vi "PH_Calorimeter_USB.ProcCases.vi"(0 "i ref in":refnum<vi>, 1 "selector":string, 2 "Data":T1, 3 "call cluster":T2={"Object"="", "Selector"="", "CallType"=enum."synchronous", "Async Object"="", "Async Selector"="", "Data Descriptor"="", "Data"=[], "Error #"=0, "Expire"=0}, 5 "error in (no error)":errorcluster) -> (14 "i ref out":refnum<vi>, 17 "answer cluster":T2={"Object"="", "Selector"="", "CallType"=enum."synchronous", "Async Object"="", "Async Selector"="", "Data Descriptor"="", "Data"=[], "Error #"=0, "Expire"=0}, 19 "error out":errorcluster)   [LabVIEW 2014, in "PH_Calorimeter_USB.lvlib"]
doc: "This method is called by a process from within the default case in the event loop. The methods of a class that are linked to events will be called from THIS method. Add your code here."
uses:
  PH_Calorimeter_USB.lvlib
  CSCore/CSSystem/CoreDefs/CoreDefs.call_type.ctl
  CSCore/BaseProcess/BaseProcess.descriptor string definition.ctl
  CSCore/CSSystem/CoreDefs/CoreDefs.rawDataType.ctl
  PH_Calorimeter_USB.Calorimeter Settings.ctl
  PH_Calorimeter_USB.Trigger Settings.ctl
  PH_Calorimeter_USB.Calorimeter Calibration Settings.ctl
  CSCore/CSSystem/CoreLib/CoreLib.byte array 2 string.vi
  CSCore/CSSystem/CoreLib/CoreLib.string 2 byte array.vi
  CSCore/CSSystem/CoreLib/CoreLib.byte array 2 double.vi
  CSCore/CSSystem/CoreLib/CoreLib.byte array 2 int.vi
  CSCore/CSSystem/CoreLib/CoreLib.lvlib
  CSCore/BaseProcess/BaseProcess.lvlib
  PH_PSDBWriter/PH_PSDBWriter.lvlib
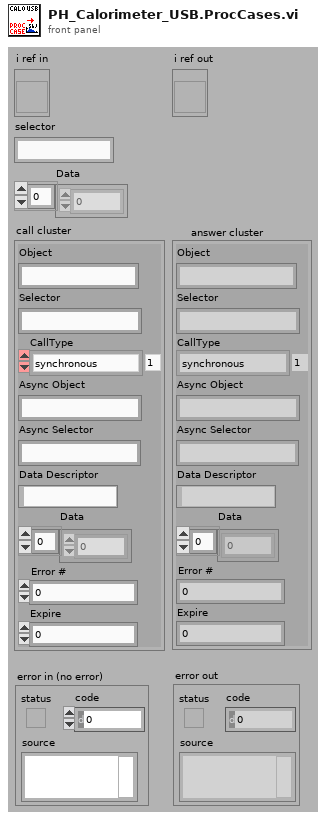
[diagram p1: front panel]
types:
  T1 = typedef "CoreDefs.rawDataType.ctl" = i8[]
  T2 = typedef "CoreDefs.call_type.ctl" = cluster{"Object":string, "Selector":string, "CallType":enum16{"simple", "synchronous", "asynchronous"}, "Async Object":string, "Async Selector":string, "Data Descriptor":T3, "Data":T1, "Error #":i32, "Expire":u32}
  T3 = typedef "BaseProcess.lvlib/BaseProcess.descriptor string definition.ctl" = string
  T4 = typedef "PH_Calorimeter_USB.lvlib/PH_Calorimeter_USB.Calorimeter Settings.ctl" = cluster{"Channel":tag, "Min Value [V]":dbl, "Max Value  [V]":dbl}
  T5 = typedef "PH_Calorimeter_USB.lvlib/PH_Calorimeter_USB.Trigger Settings.ctl" = cluster{"Channel":tag, "Min Value [V]":dbl, "Max Value  [V]":dbl, "Level [V]":dbl, "Wait Time [s]":dbl, "Length [Samples]":i32}
  T6 = typedef "PH_Calorimeter_USB.lvlib/PH_Calorimeter_USB.Calorimeter Calibration Settings.ctl" = cluster{"T 1/e [s]":dbl, "Sensitivity  [Vs/J]":dbl}
  T7 = typedef "PH_Calorimeter_USB.lvlib/PH_Calorimeter_USB.i attribute.ctl" = cluster{"GUI Refs":cluster{"Delete":refnum<vi>, "Start":refnum<vi>, "Energy":refnum<vi>, "Calorimeter":refnum<vi>, "Trigger":refnum<vi>, "Calo Calibration":refnum<vi>, "Time Base":refnum<vi>, "Device":refnum<vi>, "Graph Raw Data":refnum<vi>, "Graph Result":refnum<vi>}, "DAQ Instance":string, "Data":dbl[][], "Controller Instance":string, "Energy [J]":dbl, "Calorimeter":T4, "Trigger":T5, "Time Base":T8, "Calo Calibration":T6, "Serial Number":string}
  T8 = typedef "PH_Calorimeter_USB.lvlib/PH_Calorimeter_USB.Time Base Settings.ctl" = cluster{"Samples per Channel":i32, "Rate [Hz]":i32}
  T9 = typedef "PH_PSDBWriter.lvlib/PH_PSDBWriter.i attribute.ctl" = cluster{"PSDB Status Service ID":i32, "Instance ID":i32, "Shot #":i32, "Subsystem":T10, "Data Status":T11, "Ref PSDB Status":refnum<vi>, "PSDB Error Code":i32, "PSDB Dataset":T12, "PSDB Thread":cluster{"Ref":refnum<vi>, "Q-Ref":refnum<queue>}, "PSDB Credentials":T20}
  T10 = typedef "PH_PSDBWriter.lvlib/PH_PSDBWriter.PHELIX-Subsystems.ctl" = i32
  T11 = typedef "PH_PSDBWriter.lvlib/PH_PSDBWriter.Data Status.ctl" = i16
  T12 = typedef "PH_PSDBWriter.lvlib/PH_PSDBWriter.PSDB Dataset.ctl" = cluster{"Version":i32, "2D data Input":T13[], "Boolean Input":T15[], "Image Input":T16[], "Numeric Input":T18[], "String Input":T19[]}
  T13 = typedef "PH_PSDBWriter.lvlib/PH_PSDBWriter.2D dataset.ctl" = cluster{"name":string, "data":dbl[][], "axis description":T14}
  T14 = typedef "PSDB.lvlib/PSDB_AxisDescription.ctl" = cluster{"x axis label":string, "y axis label":string, "x axis unit":string, "y axis unit":string}
  T15 = typedef "PH_PSDBWriter.lvlib/PH_PSDBWriter.Boolean dataset.ctl" = cluster{"name":string, "data":bool, "unit":string}
  T16 = typedef "PH_PSDBWriter.lvlib/PH_PSDBWriter.Image dataset.ctl" = cluster{"name":string, "data":T17, "unit":string}
  T17 = typedef "IMAQ Image.ctl" = refnum<image>
  T18 = typedef "PH_PSDBWriter.lvlib/PH_PSDBWriter.Numeric dataset.ctl" = cluster{"name":string, "data":dbl, "unit":string}
  T19 = typedef "PH_PSDBWriter.lvlib/PH_PSDBWriter.String dataset.ctl" = cluster{"name":string, "data":string, "unit":string}
  T20 = typedef "PH_Common.lvlib/PH_Connection.PSDB Credentials.ctl" = cluster{"PW":string, "ID":string, "DS":string}
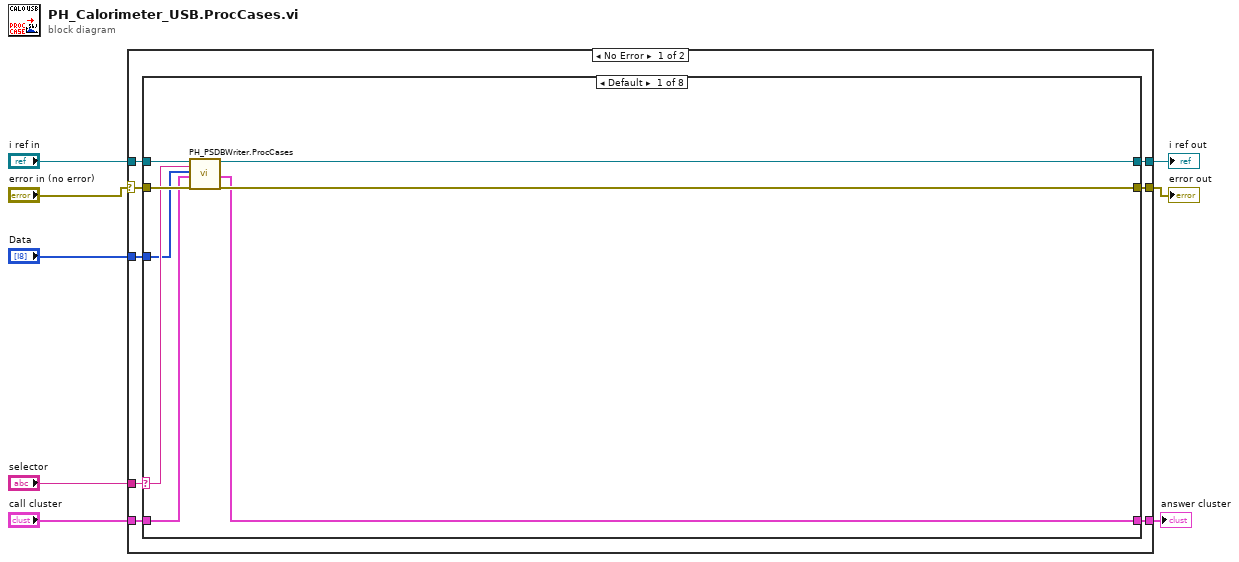
[diagram p0: block diagram]
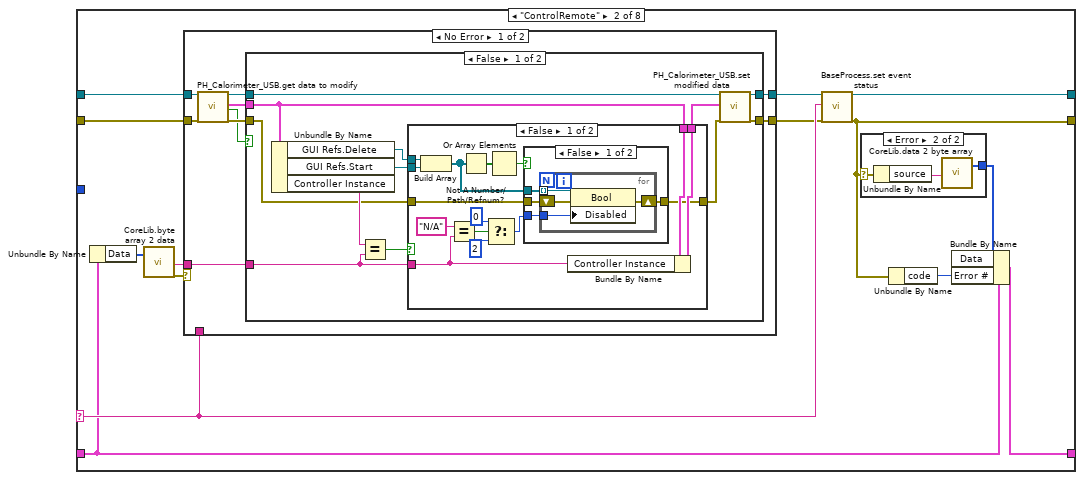
[diagram p2: hidden frame]
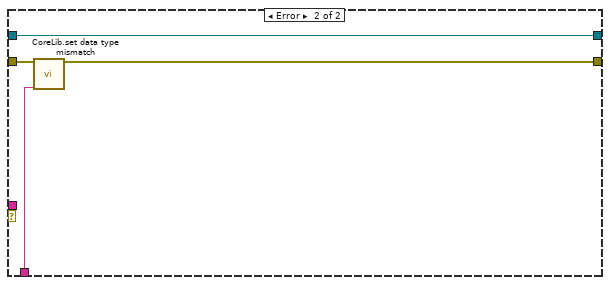
[diagram p7: hidden frame]
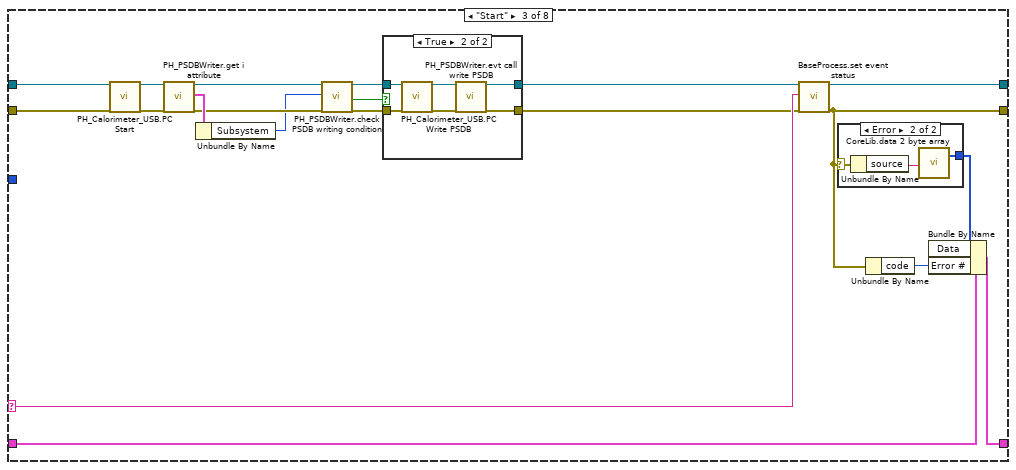
[diagram p8: hidden frame]
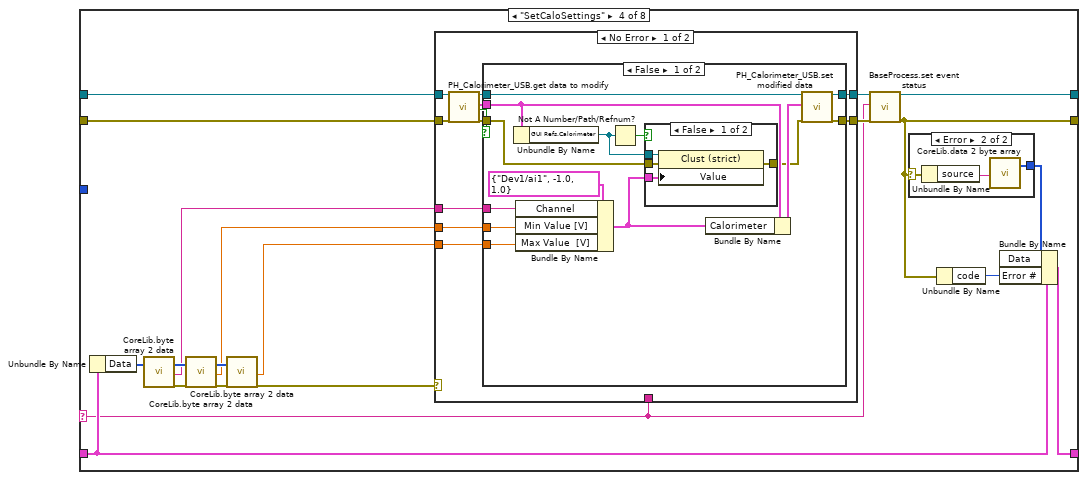
[diagram p11: hidden frame]
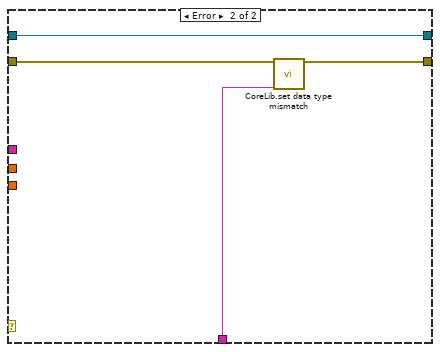
[diagram p15: hidden frame]
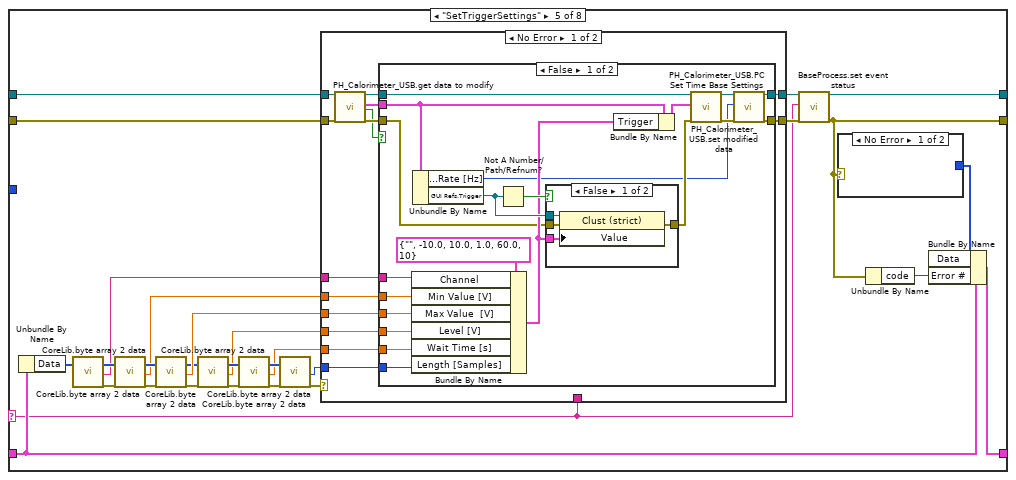
[diagram p16: hidden frame]
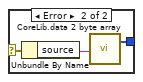
[diagram p17: hidden frame]
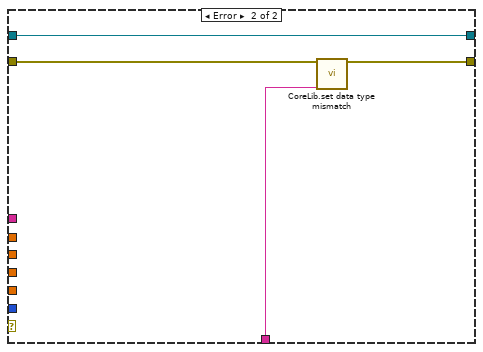
[diagram p20: hidden frame]
diagram:
  n1 = case shown="No Error" "error in (no error)" {
    selector: "error in (no error)" -> [w9 w359]
    tunnel: "selector" -> [w16 _]
    tunnel: [w15 w358] -> w7
    tunnel: "call cluster" -> [w14 w358]
    tunnel: "i ref in" -> [w13 w360]
    tunnel: [w12 w360] -> w4
    tunnel: [w11 w359] -> w3
    tunnel: "Data" -> [w10 _]
    frame No Error {
      n2 = case shown="Default" w16 {
        selector: w16 -> [w19 w31 w109 w135 w203 w269 w323 w349]
        tunnel: w13 -> [w18 w38 w107 w145 w213 w278 w332 w346]
        tunnel: [w24 w28 w112 w138 w206 w272 w326 w351] -> w12
        tunnel: w14 -> [w20 w26 w110 w136 w204 w270 w324 w348]
        tunnel: [w21 w25 w108 w134 w202 w268 w322 w347] -> w15
        tunnel: w9 -> [w23 w37 w106 w144 w212 w277 w331 w345]
        tunnel: [w22 w27 w111 w137 w205 w271 w325 w350] -> w11
        tunnel: w10 -> [w17 _ _ _ _ _ _ _]
        frame Default {
          n3 = call "PH_PSDBWriter.ProcCases.vi"("i ref in"=w18, "selector"=w19, "Data"=w17, "call cluster"=w20, "error in"=w23) -> ("i ref out"=w24:refnum<vi>, "answer cluster"=w21:T2, "error out"=w22:errorcluster)  [unwired: 12 in]
        }
        frame "ControlRemote" {
          n4 = Unbundle By Name(w26) -> ("Data"=w36:T1)
          n5 = call-poly "CoreLib.byte array 2 data.vi"("byteArray"=w36) -> ("string"=w35:string, "error out"=w34:errorcluster)  [unwired: 16 in, 1 out]
          n6 = case shown="No Error" w34 {
            tunnel: [w48 w94] -> w30
            tunnel: w38 -> [w49 w94]
            tunnel: w37 -> [w47 w93]
            tunnel: [w46 w92] -> w29
            tunnel: w31 -> [_ w91]
            tunnel: w35 -> [w42 _]
            frame No Error {
              n7 = call "PH_Calorimeter_USB.get data to modify.vi"("i ref in"=w49, "error in (no error)"=w47) -> ("i ref out"=w50:refnum<vi>, "i attribute"=w43:T7, "timed out"=w44:bool, "error out"=w45:errorcluster)  [unwired: 14 in]
              n8 = case shown="False" w44 {
                tunnel: w50 -> [w62 w90]
                tunnel: [w61 w90] -> w48
                tunnel: [w60 w89] -> w46
                tunnel: w45 -> [w52 w89]
                tunnel: w43 -> [w58 _]
                tunnel: w42 -> [w55 _]
                frame False {
                  n9 = Unbundle By Name(w58) -> ("GUI Refs.Delete"=w54:refnum<vi>, "GUI Refs.Start"=w53:refnum<vi>, "Controller Instance"=w57:string)
                  n10 = Equal?(x=w57, y=w55) -> (x = y?=w56:bool)
                  n11 = case shown="False" w56 {
                    tunnel: [w77 w88] -> w59
                    tunnel: w58 -> [w76 w88]
                    tunnel: w55 -> [w71 _]
                    tunnel: w54 -> [w74 _]
                    tunnel: w53 -> [w75 _]
                    tunnel: w52 -> [w64 w87]
                    tunnel: [w63 w87] -> w51
                    frame False {
                      n12 = Build Array(w74, w75) -> (w69:refnum<vi>[])
                      n13 = Equal?(x="N/A", y=w71) -> (x = y?=w68:bool)
                      n14 = Not A Number/Path/Refnum?(number/path/refnum=w69) -> (NaN/Path/Refnum?=w73:bool[])
                      n15 = Select(t=0, s=w68, f=2) -> (s? t:f=w67:i32)
                      n16 = Or Array Elements(Boolean array=w73) -> (logical OR=w72:bool)
                      n17 = case shown="False" w72 {
                        tunnel: w69 -> [w81 _]
                        tunnel: w67 -> [w80 _]
                        tunnel: w64 -> [w79 w86]
                        tunnel: [w78 w86] -> w63
                        frame False {
                          n18 = for {
                            tunnel: w81 -> [w85] mode=indexing
                            tunnel: w80 -> [w84]
                            shift-right: [w82] -> w78
                            shift-left: w79 -> [w83]
                            n19 = property class="Bool"(reference=w85, error in=w83, "Disabled"=w84) -> (error out=w82:errorcluster)  [unwired: 1 out]
                          }
                        }
                        frame True {
                        }
                      }
                      n20 = Bundle By Name(cluster=w76, "Controller Instance"=w71) -> (w77:T7)
                    }
                    frame True {
                    }
                  }
                  n21 = call "PH_Calorimeter_USB.set modified data.vi"("i ref in"=w62, "i attribute"=w59, "error in (no error)"=w51) -> ("i ref out"=w61:refnum<vi>, "error out"=w60:errorcluster)  [unwired: 15 in]
                }
                frame True {
                }
              }
            }
            frame Error {
              n22 = call "CoreLib.set data type mismatch.vi"("error in (no error)"=w93, "error source"=w91) -> ("error out"=w92:errorcluster)  [unwired: 17 in]
            }
          }
          n23 = call "BaseProcess.set event status.vi"("i ref in"=w30, "EventStatus"=w31, "error in (no error)"=w29) -> ("i ref out"=w28:refnum<vi>, "error out"=w27:errorcluster)  [unwired: 14 in, 1 out]
          n24 = case shown="Error" w27 {
            selector: w27 -> [_ w41]
            tunnel: [_ w39] -> w33
            frame No Error {
            }
            frame Error {
              n25 = Unbundle By Name(w41) -> ("source"=w40:string)
              n26 = call-poly "CoreLib.data 2 byte array.vi"("string"=w40) -> ("byteArray out"=w39:T1)  [unwired: 18 in]
            }
          }
          n27 = Unbundle By Name(w27) -> ("code"=w32:i32)
          n28 = Bundle By Name(cluster=w26, "Data"=w33, "Error #"=w32) -> (w25:T2)
        }
        frame "Start" {
          n29 = call "PH_Calorimeter_USB.PC Start.vi"("i ref in"=w107, "error in (no error)"=w106) -> ("i ref out"=w104:refnum<vi>, "error out"=w105:errorcluster)  [unwired: 16 in]
          n30 = call "PH_PSDBWriter.get i attribute.vi"("i ref in"=w104, "error in (no error)"=w105) -> ("i ref out"=w98:refnum<vi>, "i attribute"=w103:T9, "error out"=w102:errorcluster)  [unwired: 15 in]
          n31 = Unbundle By Name(w103) -> ("Subsystem"=w96:T10)
          n32 = call "PH_PSDBWriter.check PSDB writing condition.vi"("i ref in"=w98, "wanted Subsystem"=w96, "error IO"=w102) -> ("i ref out"=w97:refnum<vi>, "write PSDB?"=w95:bool, "error out"=w99:errorcluster)  [unwired: 14 in]
          n33 = case shown="True" w95 {
            tunnel: [w115 w122] -> w101
            tunnel: [w116 w121] -> w100
            tunnel: w99 -> [w115 w118]
            tunnel: w97 -> [w116 w117]
            frame False {
            }
            frame True {
              n34 = call "PH_Calorimeter_USB.PC Write PSDB.vi"("i ref in"=w117, "error IO"=w118) -> ("i ref out"=w119:refnum<vi>, "error out"=w120:errorcluster)  [unwired: 16 in]
              n35 = call "PH_PSDBWriter.evt call write PSDB.vi"("i ref in"=w119, "error in (no error)"=w120) -> ("i ref out"=w121:refnum<vi>, "error out"=w122:errorcluster)  [unwired: 16 in]
            }
          }
          n36 = call "BaseProcess.set event status.vi"("i ref in"=w100, "EventStatus"=w109, "error in (no error)"=w101) -> ("i ref out"=w112:refnum<vi>, "error out"=w111:errorcluster)  [unwired: 14 in, 1 out]
          n37 = case shown="Error" w111 {
            selector: w111 -> [_ w125]
            tunnel: [_ w123] -> w114
            frame No Error {
            }
            frame Error {
              n38 = Unbundle By Name(w125) -> ("source"=w124:string)
              n39 = call-poly "CoreLib.data 2 byte array.vi"("string"=w124) -> ("byteArray out"=w123:T1)  [unwired: 18 in]
            }
          }
          n40 = Unbundle By Name(w111) -> ("code"=w113:i32)
          n41 = Bundle By Name(cluster=w110, "Data"=w114, "Error #"=w113) -> (w108:T2)
        }
        frame "SetCaloSettings" {
          n42 = Unbundle By Name(w136) -> ("Data"=w143:T1)
          n43 = call-poly "CoreLib.byte array 2 data.vi"("byteArray"=w143) -> ("byteArray out"=w130:T1, "string"=w128:string, "error out"=w133:errorcluster)  [unwired: 16 in]
          n44 = call-poly "CoreLib.byte array 2 data.vi"("byteArray"=w130, "error in (no error)"=w133) -> ("byteArray out"=w129:T1, "d64"=w127:dbl, "error out"=w132:errorcluster)  [unwired: 15 in]
          n45 = call-poly "CoreLib.byte array 2 data.vi"("byteArray"=w129, "error in (no error)"=w132) -> ("d64"=w126:dbl, "error out"=w131:errorcluster)  [unwired: 15 in, 1 out]
          n46 = case shown="No Error" w131 {
            tunnel: [w156 w184] -> w139
            tunnel: w145 -> [w159 w184]
            tunnel: w144 -> [w158 w183]
            tunnel: [w154 w182] -> w140
            tunnel: w135 -> [_ w181]
            tunnel: w128 -> [w151 _]
            tunnel: w127 -> [w150 _]
            tunnel: w126 -> [w149 _]
            frame No Error {
              n47 = call "PH_Calorimeter_USB.get data to modify.vi"("i ref in"=w159, "error in (no error)"=w158) -> ("i ref out"=w157:refnum<vi>, "i attribute"=w153:T7, "timed out"=w152:bool, "error out"=w155:errorcluster)  [unwired: 14 in]
              n48 = case shown="False" w152 {
                tunnel: w157 -> [w173 w180]
                tunnel: [w172 w180] -> w156
                tunnel: w155 -> [w161 w179]
                tunnel: [w171 w179] -> w154
                tunnel: w153 -> [w169 _]
                tunnel: w151 -> [w164 _]
                tunnel: w150 -> [w163 _]
                tunnel: w149 -> [w162 _]
                frame False {
                  n49 = Unbundle By Name(w169) -> ("GUI Refs.Calorimeter"=w168:refnum<vi>)
                  n50 = Bundle By Name(cluster=T4 {"Channel"="Dev1/ai1", "Min Value [V]"=-1.0, "Max Value  [V]"=1.0} ("Calorimeter"), "Channel"=w164, "Min Value [V]"=w163, "Max Value  [V]"=w162) -> (w165:T4)
                  n51 = Not A Number/Path/Refnum?(number/path/refnum=w168) -> (NaN/Path/Refnum?=w167:bool)
                  n52 = case shown="False" w167 {
                    tunnel: w161 -> [w177 w178]
                    tunnel: w168 -> [w176 _]
                    tunnel: w165 -> [w175 _]
                    tunnel: [w174 w178] -> w160
                    frame False {
                      n53 = property class="Clust (strict)"(reference=w176, error in=w177, "Value"=w175) -> (error out=w174:errorcluster)  [unwired: 1 out]
                    }
                    frame True {
                    }
                  }
                  n54 = Bundle By Name(cluster=w169, "Calorimeter"=w165) -> (w170:T7)
                  n55 = call "PH_Calorimeter_USB.set modified data.vi"("i ref in"=w173, "i attribute"=w170, "error in (no error)"=w160) -> ("i ref out"=w172:refnum<vi>, "error out"=w171:errorcluster)  [unwired: 15 in]
                }
                frame True {
                }
              }
            }
            frame Error {
              n56 = call "CoreLib.set data type mismatch.vi"("error in (no error)"=w183, "error source"=w181) -> ("error out"=w182:errorcluster)  [unwired: 17 in]
            }
          }
          n57 = call "BaseProcess.set event status.vi"("i ref in"=w139, "EventStatus"=w135, "error in (no error)"=w140) -> ("i ref out"=w138:refnum<vi>, "error out"=w137:errorcluster)  [unwired: 14 in, 1 out]
          n58 = case shown="Error" w137 {
            selector: w137 -> [_ w148]
            tunnel: [_ w146] -> w142
            frame No Error {
            }
            frame Error {
              n59 = Unbundle By Name(w148) -> ("source"=w147:string)
              n60 = call-poly "CoreLib.data 2 byte array.vi"("string"=w147) -> ("byteArray out"=w146:T1)  [unwired: 18 in]
            }
          }
          n61 = Unbundle By Name(w137) -> ("code"=w141:i32)
          n62 = Bundle By Name(cluster=w136, "Data"=w142, "Error #"=w141) -> (w134:T2)
        }
        frame "SetTriggerSettings" {
          n63 = Unbundle By Name(w204) -> ("Data"=w211:T1)
          n64 = call-poly "CoreLib.byte array 2 data.vi"("byteArray"=w211) -> ("byteArray out"=w199:T1, "string"=w197:string, "error out"=w201:errorcluster)  [unwired: 16 in]
          n65 = call-poly "CoreLib.byte array 2 data.vi"("byteArray"=w199, "error in (no error)"=w201) -> ("byteArray out"=w198:T1, "d64"=w196:dbl, "error out"=w200:errorcluster)  [unwired: 15 in]
          n66 = call-poly "CoreLib.byte array 2 data.vi"("byteArray"=w198, "error in (no error)"=w200) -> ("byteArray out"=w188:T1, "d64"=w195:dbl, "error out"=w191:errorcluster)  [unwired: 15 in]
          n67 = call-poly "CoreLib.byte array 2 data.vi"("byteArray"=w188, "error in (no error)"=w191) -> ("byteArray out"=w193:T1, "d64"=w189:dbl, "error out"=w194:errorcluster)  [unwired: 15 in]
          n68 = call-poly "CoreLib.byte array 2 data.vi"("byteArray"=w193, "error in (no error)"=w194) -> ("byteArray out"=w187:T1, "d64"=w186:dbl, "error out"=w192:errorcluster)  [unwired: 15 in]
          n69 = call-poly "CoreLib.byte array 2 data.vi"("byteArray"=w187, "error in (no error)"=w192) -> ("i32"=w185:i32, "error out"=w190:errorcluster)  [unwired: 15 in, 1 out]
          n70 = case shown="No Error" w190 {
            tunnel: [w227 w261] -> w207
            tunnel: w213 -> [w230 w261]
            tunnel: w212 -> [w229 w260]
            tunnel: [w225 w259] -> w208
            tunnel: w203 -> [_ w258]
            tunnel: w197 -> [w222 _]
            tunnel: w196 -> [w221 _]
            tunnel: w195 -> [w220 _]
            tunnel: w189 -> [w219 _]
            tunnel: w186 -> [w218 _]
            tunnel: w185 -> [w217 _]
            frame No Error {
              n71 = call "PH_Calorimeter_USB.get data to modify.vi"("i ref in"=w230, "error in (no error)"=w229) -> ("i ref out"=w228:refnum<vi>, "i attribute"=w224:T7, "timed out"=w223:bool, "error out"=w226:errorcluster)  [unwired: 14 in]
              n72 = case shown="False" w223 {
                tunnel: w228 -> [w250 w257]
                tunnel: [w234 w257] -> w227
                tunnel: w226 -> [w236 w256]
                tunnel: [w232 w256] -> w225
                tunnel: w224 -> [w248 _]
                tunnel: w222 -> [w245 _]
                tunnel: w221 -> [w244 _]
                tunnel: w220 -> [w243 _]
                tunnel: w219 -> [w240 _]
                tunnel: w218 -> [w237 _]
                tunnel: w217 -> [w239 _]
                frame False {
                  n73 = Bundle By Name(cluster=T5 {"Channel"="", "Min Value [V]"=-10.0, "Max Value  [V]"=10.0, "Level [V]"=1.0, "Wait Time [s]"=60.0, "Length [Samples]"=10} ("Trigger"), "Channel"=w245, "Min Value [V]"=w244, "Max Value  [V]"=w243, "Level [V]"=w240, "Wait Time [s]"=w237, "Length [Samples]"=w239) -> (w238:T5)
                  n74 = Unbundle By Name(w248) -> ("Time Base.Rate [Hz]"=w231:i32, "GUI Refs.Trigger"=w247:refnum<vi>)
                  n75 = Not A Number/Path/Refnum?(number/path/refnum=w247) -> (NaN/Path/Refnum?=w246:bool)
                  n76 = case shown="False" w246 {
                    tunnel: w236 -> [w254 w255]
                    tunnel: w247 -> [w253 _]
                    tunnel: w238 -> [w252 _]
                    tunnel: [w251 w255] -> w242
                    frame False {
                      n77 = property class="Clust (strict)"(reference=w253, error in=w254, "Value"=w252) -> (error out=w251:errorcluster)  [unwired: 1 out]
                    }
                    frame True {
                    }
                  }
                  n78 = Bundle By Name(cluster=w248, "Trigger"=w238) -> (w249:T7)
                  n79 = call "PH_Calorimeter_USB.set modified data.vi"("i ref in"=w250, "i attribute"=w249, "error in (no error)"=w242) -> ("i ref out"=w235:refnum<vi>, "error out"=w233:errorcluster)  [unwired: 15 in]
                  n80 = call "PH_Calorimeter_USB.PC Set Time Base Settings.vi"("i ref in"=w235, "Rate [Hz]"=w231, "error in (no error)"=w233) -> ("i ref out"=w234:refnum<vi>, "error out"=w232:errorcluster)  [unwired: 15 in]
                }
                frame True {
                }
              }
            }
            frame Error {
              n81 = call "CoreLib.set data type mismatch.vi"("error in (no error)"=w260, "error source"=w258) -> ("error out"=w259:errorcluster)  [unwired: 17 in]
            }
          }
          n82 = call "BaseProcess.set event status.vi"("i ref in"=w207, "EventStatus"=w203, "error in (no error)"=w208) -> ("i ref out"=w206:refnum<vi>, "error out"=w205:errorcluster)  [unwired: 14 in, 1 out]
          n83 = case shown="No Error" w205 {
            selector: w205 -> [_ w216]
            tunnel: [_ w214] -> w210
            frame No Error {
            }
            frame Error {
              n84 = Unbundle By Name(w216) -> ("source"=w215:string)
              n85 = call-poly "CoreLib.data 2 byte array.vi"("string"=w215) -> ("byteArray out"=w214:T1)  [unwired: 18 in]
            }
          }
          n86 = Unbundle By Name(w205) -> ("code"=w209:i32)
          n87 = Bundle By Name(cluster=w204, "Data"=w210, "Error #"=w209) -> (w202:T2)
        }
        frame "SetCaloCalibrationSettings" {
          n88 = Unbundle By Name(w270) -> ("Data"=w263:T1)
          n89 = call-poly "CoreLib.byte array 2 data.vi"("byteArray"=w263) -> ("byteArray out"=w266:T1, "d64"=w265:dbl, "error out"=w267:errorcluster)  [unwired: 16 in]
          n90 = call-poly "CoreLib.byte array 2 data.vi"("byteArray"=w266, "error in (no error)"=w267) -> ("d64"=w264:dbl, "error out"=w262:errorcluster)  [unwired: 15 in, 1 out]
          n91 = case shown="No Error" w262 {
            tunnel: [w288 w318] -> w273
            tunnel: w278 -> [w291 w318]
            tunnel: w277 -> [w290 w317]
            tunnel: [w286 w316] -> w274
            tunnel: w269 -> [_ w315]
            tunnel: w265 -> [w283 _]
            tunnel: w264 -> [w282 _]
            frame No Error {
              n92 = call "PH_Calorimeter_USB.get data to modify.vi"("i ref in"=w291, "error in (no error)"=w290) -> ("i ref out"=w289:refnum<vi>, "i attribute"=w285:T7, "timed out"=w284:bool, "error out"=w287:errorcluster)  [unwired: 14 in]
              n93 = case shown="False" w284 {
                tunnel: w289 -> [w307 w314]
                tunnel: [w295 w314] -> w288
                tunnel: w287 -> [w301 w313]
                tunnel: [w293 w313] -> w286
                tunnel: w285 -> [w305 _]
                tunnel: w283 -> [w297 _]
                tunnel: w282 -> [w302 _]
                frame False {
                  n94 = Unbundle By Name(w305) -> ("Time Base.Rate [Hz]"=w292:i32, "GUI Refs.Calo Calibration"=w304:refnum<vi>)
                  n95 = Bundle By Name(cluster=T6 {"T 1/e [s]"=220.0, "Sensitivity  [Vs/J]"=0.0592} ("Calo Calibration"), "T 1/e [s]"=w297, "Sensitivity  [Vs/J]"=w302) -> (w299:T6)
                  n96 = Not A Number/Path/Refnum?(number/path/refnum=w304) -> (NaN/Path/Refnum?=w303:bool)
                  n97 = case shown="False" w303 {
                    tunnel: w301 -> [w311 w312]
                    tunnel: w304 -> [w310 _]
                    tunnel: w299 -> [w309 _]
                    tunnel: [w308 w312] -> w300
                    frame False {
                      n98 = property class="Clust (strict)"(reference=w310, error in=w311, "Value"=w309) -> (error out=w308:errorcluster)  [unwired: 1 out]
                    }
                    frame True {
                    }
                  }
                  n99 = Bundle By Name(cluster=w305, "Calo Calibration"=w299) -> (w306:T7)
                  n100 = call "PH_Calorimeter_USB.set modified data.vi"("i ref in"=w307, "i attribute"=w306, "error in (no error)"=w300) -> ("i ref out"=w296:refnum<vi>, "error out"=w294:errorcluster)  [unwired: 15 in]
                  n101 = call "PH_Calorimeter_USB.PC Set Time Base Settings.vi"("i ref in"=w296, "Rate [Hz]"=w292, "error in (no error)"=w294) -> ("i ref out"=w295:refnum<vi>, "error out"=w293:errorcluster)  [unwired: 15 in]
                }
                frame True {
                }
              }
            }
            frame Error {
              n102 = call "CoreLib.set data type mismatch.vi"("error in (no error)"=w317, "error source"=w315) -> ("error out"=w316:errorcluster)  [unwired: 17 in]
            }
          }
          n103 = call "BaseProcess.set event status.vi"("i ref in"=w273, "EventStatus"=w269, "error in (no error)"=w274) -> ("i ref out"=w272:refnum<vi>, "error out"=w271:errorcluster)  [unwired: 14 in, 1 out]
          n104 = case shown="No Error" w271 {
            selector: w271 -> [_ w281]
            tunnel: [_ w279] -> w276
            frame No Error {
            }
            frame Error {
              n105 = Unbundle By Name(w281) -> ("source"=w280:string)
              n106 = call-poly "CoreLib.data 2 byte array.vi"("string"=w280) -> ("byteArray out"=w279:T1)  [unwired: 18 in]
            }
          }
          n107 = Unbundle By Name(w271) -> ("code"=w275:i32)
          n108 = Bundle By Name(cluster=w270, "Data"=w276, "Error #"=w275) -> (w268:T2)
        }
        frame "SetTimeBaseSettings" {
          n109 = Unbundle By Name(w324) -> ("Data"=w319:T1)
          n110 = call-poly "CoreLib.byte array 2 data.vi"("byteArray"=w319) -> ("i32"=w320:i32, "error out"=w321:errorcluster)  [unwired: 16 in, 1 out]
          n111 = case shown="No Error" w321 {
            tunnel: [w338 w344] -> w327
            tunnel: w332 -> [w340 w344]
            tunnel: w331 -> [w339 w343]
            tunnel: [w337 w342] -> w328
            tunnel: w323 -> [_ w341]
            tunnel: w320 -> [w336 _]
            frame No Error {
              n112 = call "PH_Calorimeter_USB.PC Set Time Base Settings.vi"("i ref in"=w340, "Rate [Hz]"=w336, "error in (no error)"=w339) -> ("i ref out"=w338:refnum<vi>, "error out"=w337:errorcluster)  [unwired: 15 in]
            }
            frame Error {
              n113 = call "CoreLib.set data type mismatch.vi"("error in (no error)"=w343, "error source"=w341) -> ("error out"=w342:errorcluster)  [unwired: 17 in]
            }
          }
          n114 = call "BaseProcess.set event status.vi"("i ref in"=w327, "EventStatus"=w323, "error in (no error)"=w328) -> ("i ref out"=w326:refnum<vi>, "error out"=w325:errorcluster)  [unwired: 14 in, 1 out]
          n115 = case shown="Error" w325 {
            selector: w325 -> [_ w335]
            tunnel: [_ w333] -> w330
            frame No Error {
            }
            frame Error {
              n116 = Unbundle By Name(w335) -> ("source"=w334:string)
              n117 = call-poly "CoreLib.data 2 byte array.vi"("string"=w334) -> ("byteArray out"=w333:T1)  [unwired: 18 in]
            }
          }
          n118 = Unbundle By Name(w325) -> ("code"=w329:i32)
          n119 = Bundle By Name(cluster=w324, "Data"=w330, "Error #"=w329) -> (w322:T2)
        }
        frame "_set_PSDB_Data" {
          n120 = call "BaseProcess.set event status.vi"("i ref in"=w346, "EventStatus"=w349, "error in (no error)"=w345) -> ("i ref out"=w351:refnum<vi>, "error out"=w350:errorcluster)  [unwired: 14 in, 1 out]
          n121 = case shown="No Error" w350 {
            selector: w350 -> [_ w357]
            tunnel: [_ w355] -> w352
            frame No Error {
            }
            frame Error {
              n122 = Unbundle By Name(w357) -> ("source"=w356:string)
              n123 = call-poly "CoreLib.data 2 byte array.vi"("string"=w356) -> ("byteArray out"=w355:T1)  [unwired: 18 in]
            }
          }
          n124 = Unbundle By Name(w350) -> ("code"=w354:i32)
          n125 = Bundle By Name(cluster=w348, "Data"=w352, "Error #"=w354, "Data Descriptor"="C:N") -> (w347:T2)
        }
      }
    }
    frame Error {
    }
  }
  "answer cluster" <- w7
  "i ref out" <- w4
  "error out" <- w3
